vi "Stepper Step Mode Example.vi"() -> ()   [LabVIEW 2012, in "Phidget Stepper.lvlib"]
uses:
  <instrlib>/Phidgets/Phidget Stepper/Phidget Stepper.lvlib
  <instrlib>/Phidgets/Phidget Stepper/Public/StepperStart.vi
  <instrlib>/Phidgets/Phidget Stepper/Public/StepperClose.vi
  <instrlib>/Phidgets/Phidget Common/Phidget Common.lvlib
panel:
  in  "Stepper Initialization Data":T1={"Control Mode"=0, " Rescale Factor"=1.0, "Velocity Limit"=10000.0, "Acceleration"=10000.0, "Current Limit"=1.0} {"Control Mode" items=["Step", "Run"]}
  in  "Target Position":dbl
  out "Velocity":dbl
  out "Position":dbl
  out "Moving":bool
  in  "Device Info":T2={"Serial Number"=-1, "Channel"=0, "Port"=0}
  out "Attached?":bool
  out "Serial Number Return":i32
  out "error out":errorcluster
  # "NOTE: The default\nVelocity Limit and\nAcceleration\nparameters will not\nwork with the 1062.\nThese may be\nboth set to 200\n(or any other value \nin the valid range)\nfor the device to\nwork."
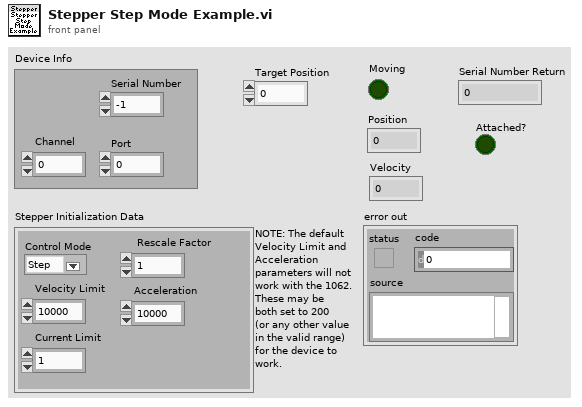
[diagram p1: front panel]
types:
  T1 = cluster{"Control Mode":u16, " Rescale Factor":dbl, "Velocity Limit":dbl, "Acceleration":dbl, "Current Limit":dbl}
  T2 = cluster{"Serial Number":i32, "Channel":i32, "Port":i32}
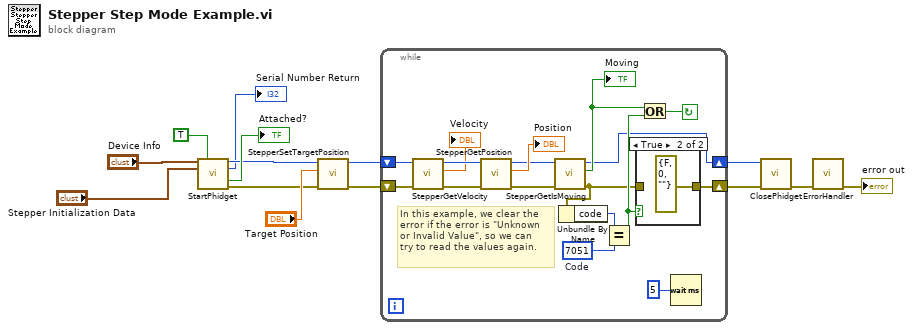
[diagram p0: block diagram]
diagram:
  n1 = call-poly <instrlib>:"StartPhidget.vi"("Device Info"="Device Info", "Engaged"=TRUE, "Stepper Initialization Data"="Stepper Initialization Data") -> ("Phidget ID"=w8:u64, "Serial Number Return"=→"Serial Number Return":i32, "Attached?"=→"Attached?":bool, "error out"=w6:errorcluster)  [unwired: 9 in]
  n2 = call <instrlib>:"StepperSetTargetPosition.vi"("error in (no error)"=w6, "Target Position Position"="Target Position", "Device In"=w8) -> ("error out"=w3:errorcluster, "Device Out"=w2:u64)  [unwired: 6 in]
  n3 = while {
    shift-right: [w15] -> w10
    shift-left: w2 -> [w24]
    shift-right: [w16] -> w11
    shift-left: w3 -> [w25]
    stop <- w19 continue-if-true
    w21 = 7051  # Code
    # "In this example, we clear the\nerror if the error is \"Unknown\nor Invalid Value\", so we can\ntry to read the values again."
    n4 = call <instrlib>:"StepperGetVelocity.vi"("error in (no error)"=w25, "Device In"=w24) -> ("error out"=w27:errorcluster, "Velocity"=→"Velocity":dbl, "Device Out"=w26:u64)  [unwired: 6 in]
    n5 = call <instrlib>:"StepperGetPosition.vi"("error in (no error)"=w27, "Device In"=w26) -> ("error out"=w28:errorcluster, "Position"=→"Position":dbl, "Device Out"=w29:u64)  [unwired: 6 in]
    n6 = call <instrlib>:"StepperGetIsMoving.vi"("error in (no error)"=w28, "Device In"=w29) -> ("error out"=w17:errorcluster, "Moving"=w20:bool, "Device Out"=w15:u64)  [unwired: 6 in]
    "Moving" <- w20
    n7 = Unbundle By Name(w17) -> ("code"=w22:i32)
    n8 = Equal?(x=w22, y=w21) -> (x = y?=w18:bool)
    n9 = case shown="True" w18 {
      tunnel: w17 -> [w32 _]
      tunnel: [w32 errorcluster {"status"=FALSE, "code"=0, "source"=""} ("error constant")] -> w16
      frame False {
      }
      frame True {
      }
    }
    n10 = Or(x=w20, y=w18) -> (x .or. y?=w19:bool)
    n11 = Wait (ms)(milliseconds to wait=u32 5) -> ()  [unwired: 1 out]
  }
  n12 = call-poly <instrlib>:"ClosePhidget.vi"("error in"=w11, "Device In"=w10) -> ("error out"=w14:errorcluster)  [unwired: 9 in]
  n13 = call <instrlib>:"ErrorHandler.vi"("error in"=w14) -> ("error out"=→"error out":errorcluster)  [unwired: 9 in, 1 out]
